vi "Tx to UDP.vi"(5 "Data Conversion":T1, 7 "Header Info":bool[](array[boolean]), 8 "error in (no error)":errorcluster, 9 "Byte Order":T4(ring), 10 "Tx Array":dbl[](array[numeric]), 11 "Packet ID":i32) -> (0 "error out":errorcluster, 2 "Tx String":string)   [LabVIEW 2016, in "UDP-Custom-Device Engine.lvlib"]
uses:
  UDP-Custom-Device Engine.lvlib
  Data Conversion Config.ctl
  <vilib>/NI Veristand/VeriStand Data/Library/Byte Buffer/Byte Buffer.lvclass
  <vilib>/NI Veristand/VeriStand Data/Library/Byte Buffer/Byte Buffer.Mapping.ctl
  <vilib>/NI Veristand/VeriStand Data/Library/Typedefs/Typedefs.Data Types.ctl
  <vilib>/NI Veristand/VeriStand Data/Library/Byte Buffer/Byte Buffer.lvclass/Byte Buffer.ctl
  <vilib>/NI Veristand/VeriStand Data/Library/Memory Management/Memory Management.MoveDblBlock.Write (Double).vi
  <vilib>/NI Veristand/VeriStand Data/Library/Byte Buffer/Byte Buffer.Write.Typed Array.vi
  <vilib>/NI Veristand/VeriStand Data/Library/Utilities/Utilities.Buffer.Double.vi
  <vilib>/NI Veristand/VeriStand Data/Library/Byte Buffer/Byte Buffer.Write.vi
  <vilib>/NI Veristand/VeriStand Data/Library/Byte Buffer/Byte Buffer.Write (1D Boolean).vi
  <vilib>/NI Veristand/VeriStand Data/Library/Type Conversion/Type Conversion.From Double.Subset.vi
  <vilib>/NI Veristand/VeriStand Data/Library/Type Conversion/Type Conversion.From Double.Subset (1D Boolean).vi
  <vilib>/NI Veristand/VeriStand Data/Library/Byte Buffer/Byte Buffer.Write (1D SGL).vi
  <vilib>/NI Veristand/VeriStand Data/Library/Type Conversion/Type Conversion.From Double.Subset (1D SGL).vi
  <vilib>/NI Veristand/VeriStand Data/Library/Byte Buffer/Byte Buffer.Write (1D DBL).vi
  <vilib>/NI Veristand/VeriStand Data/Library/Byte Buffer/Byte Buffer.Write (1D I8).vi
  <vilib>/NI Veristand/VeriStand Data/Library/Type Conversion/Type Conversion.From Double.Subset (1D I8).vi
  <vilib>/NI Veristand/VeriStand Data/Library/Byte Buffer/Byte Buffer.Write (1D I16).vi
  <vilib>/NI Veristand/VeriStand Data/Library/Type Conversion/Type Conversion.From Double.Subset (1D I16).vi
  <vilib>/NI Veristand/VeriStand Data/Library/Byte Buffer/Byte Buffer.Write (1D I32).vi
  <vilib>/NI Veristand/VeriStand Data/Library/Type Conversion/Type Conversion.From Double.Subset (1D I32).vi
  <vilib>/NI Veristand/VeriStand Data/Library/Byte Buffer/Byte Buffer.Write (1D I64).vi
  <vilib>/NI Veristand/VeriStand Data/Library/Type Conversion/Type Conversion.From Double.Subset (1D I64).vi
  <vilib>/NI Veristand/VeriStand Data/Library/Byte Buffer/Byte Buffer.Write (1D U8).vi
  <vilib>/NI Veristand/VeriStand Data/Library/Type Conversion/Type Conversion.From Double.Subset (1D U8).vi
  <vilib>/NI Veristand/VeriStand Data/Library/Byte Buffer/Byte Buffer.Write (1D U16).vi
  <vilib>/NI Veristand/VeriStand Data/Library/Type Conversion/Type Conversion.From Double.Subset (1D U16).vi
  <vilib>/NI Veristand/VeriStand Data/Library/Byte Buffer/Byte Buffer.Write (1D U32).vi
  <vilib>/NI Veristand/VeriStand Data/Library/Type Conversion/Type Conversion.From Double.Subset (1D U32).vi
  <vilib>/NI Veristand/VeriStand Data/Library/Byte Buffer/Byte Buffer.Write (1D U64).vi
  <vilib>/NI Veristand/VeriStand Data/Library/Type Conversion/Type Conversion.From Double.Subset (1D U64).vi
  <vilib>/NI Veristand/VeriStand Data/Library/Utilities/Utilities.Sizeof.Array.vi
  <vilib>/NI Veristand/VeriStand Data/Library/Type Conversion/Type Conversion.From Double.vi
  <vilib>/NI Veristand/VeriStand Data/Library/Type Conversion/Type Conversion.From Double (1D Boolean).vi
  <vilib>/NI Veristand/VeriStand Data/Library/Type Conversion/Type Conversion.From Double (1D SGL).vi
  <vilib>/NI Veristand/VeriStand Data/Library/Type Conversion/Type Conversion.From Double (1D I8).vi
  <vilib>/NI Veristand/VeriStand Data/Library/Type Conversion/Type Conversion.From Double (1D I16).vi
  <vilib>/NI Veristand/VeriStand Data/Library/Type Conversion/Type Conversion.From Double (1D I32).vi
  <vilib>/NI Veristand/VeriStand Data/Library/Type Conversion/Type Conversion.From Double (1D I64).vi
  <vilib>/NI Veristand/VeriStand Data/Library/Type Conversion/Type Conversion.From Double (1D U8).vi
  <vilib>/NI Veristand/VeriStand Data/Library/Type Conversion/Type Conversion.From Double (1D U16).vi
  <vilib>/NI Veristand/VeriStand Data/Library/Type Conversion/Type Conversion.From Double (1D U32).vi
  <vilib>/NI Veristand/VeriStand Data/Library/Type Conversion/Type Conversion.From Double (1D U64).vi
  <vilib>/NI Veristand/VeriStand Data/Library/Utilities/Utilities.Sizeof.Scalar.vi
  <vilib>/NI Veristand/VeriStand Data/Library/Memory Management/Memory Management.Handle Return.vi
  <vilib>/NI Veristand/VeriStand Data/Library/VeriStand Data.lvlib
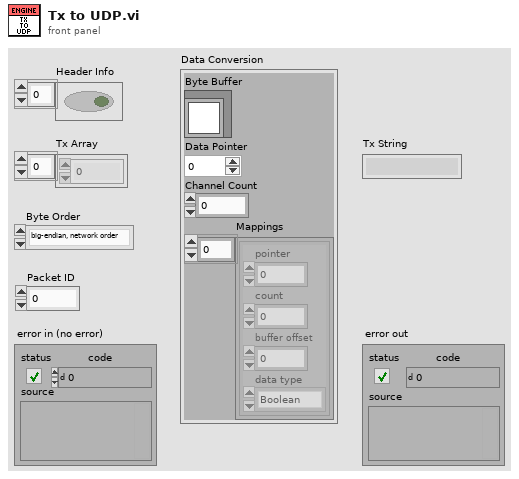
[diagram p1: front panel]
types:
  T1 = typedef "UDP-Custom-Device Engine.lvlib/Data Conversion Config.ctl" = cluster{"Byte Buffer":refnum<class "Byte Buffer.lvclass">, "Data Pointer":u64, "Channel Count":i32, "Mappings":T2[]}
  T2 = typedef "VeriStand Data.lvlib/Byte Buffer.lvclass/Byte Buffer.Mapping.ctl" = cluster{"pointer":u64, "count":i32, "buffer offset":i32, "data type":T3}
  T3 = typedef "VeriStand Data.lvlib/Typedefs.Data Types.ctl" = enum16{"Boolean", "Single", "Double", "I8", "I16", "I32", "I64", "U8", "U16", "U32", "U64"}
  T4 = enum16{"big-endian, network order", "native, host order", "little-endian"}
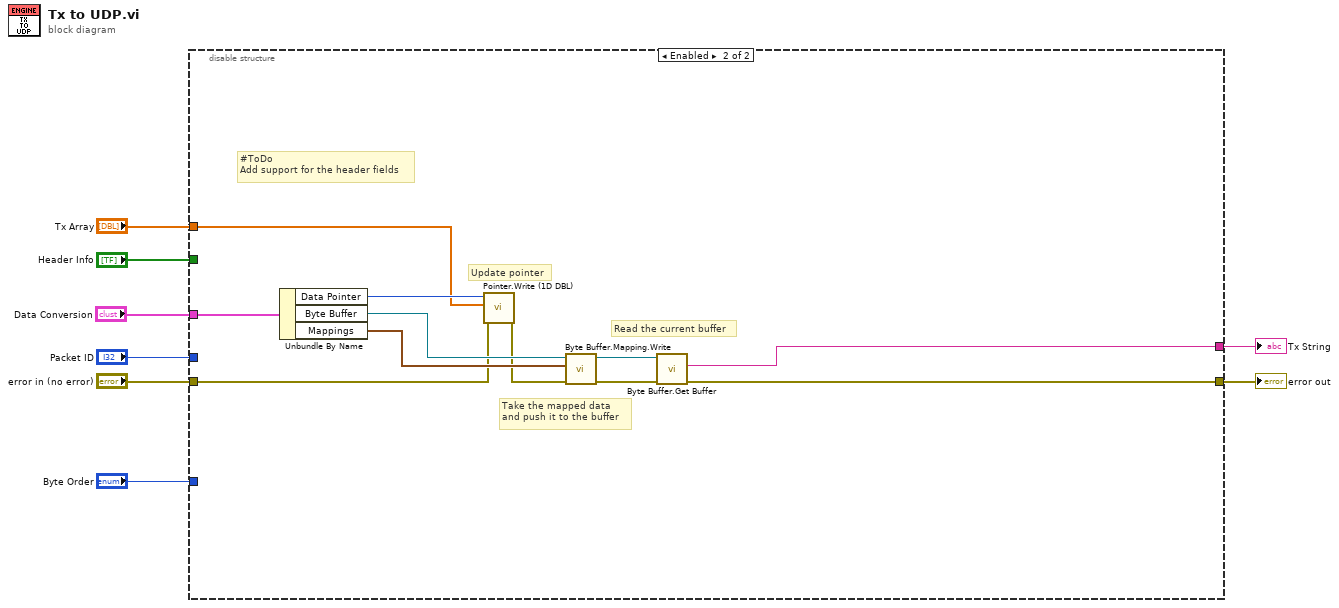
[diagram p0: block diagram]
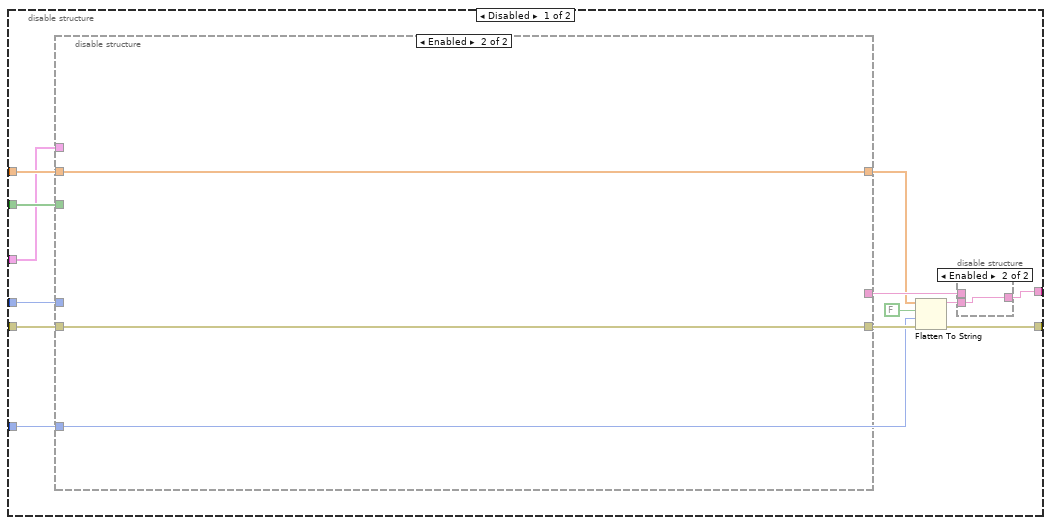
[diagram p2: hidden frame]
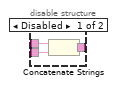
[diagram p3: hidden frame]
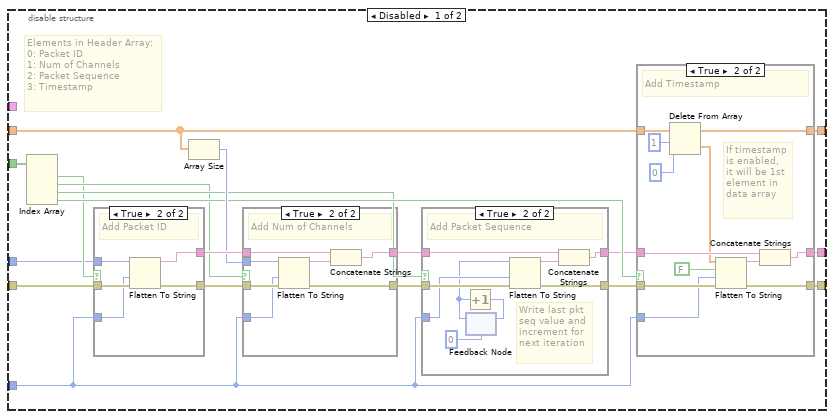
[diagram p4: hidden frame]
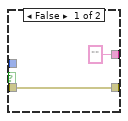
[diagram p8: hidden frame]
diagram:
  n1 = disable-structure shown="Enabled" {
    disable-tunnel: "error in (no error)" -> [w21 w94]
    disable-tunnel: [w20 w90] -> w7
    disable-tunnel: "Byte Order" -> [w16 _]
    disable-tunnel: "Header Info" -> [w15 _]
    disable-tunnel: "Tx Array" -> [w13 w97]
    disable-tunnel: "Packet ID" -> [w12 _]
    disable-tunnel: [w10 w89] -> w2
    disable-tunnel: "Data Conversion" -> [w9 w99]
    frame Disabled {
      n2 = disable-structure shown="Enabled" {
        disable-tunnel: w21 -> [w44 w87]
        disable-tunnel: [w40 w87] -> w17
        disable-tunnel: w16 -> [w38 _]
        disable-tunnel: w15 -> [w36 _]
        disable-tunnel: [w29 _] -> w14
        disable-tunnel: w13 -> [w28 w88]
        disable-tunnel: [w27 w88] -> w11
        disable-tunnel: w12 -> [w26 _]
        disable-tunnel: w9 -> [_ _]
        frame Disabled {
          # "Elements in Header Array:\n0: Packet ID\n1: Num of Channels\n2: Packet Sequence\n3: Timestamp"
          n3 = Index Array(array=w36) -> (element #1=w32:bool, element #2=w33:bool, element #3=w34:bool, element #4=w35:bool)  [unwired: 4 in]
          n4 = case shown="True" w32 {
            tunnel: w44 -> [w81 w86]
            tunnel: [w81 w85] -> w43
            tunnel: ["" ("data string") w84] -> w39
            tunnel: w38 -> [_ w83]
            tunnel: w26 -> [_ w82]
            frame False {
            }
            frame True {
              # "Add Packet ID"
              n5 = Flatten To String(anything=w82, byte order (0:big-endian, network order)=w83, error in (no error)=w86) -> (data string=w84:string, error out=w85:errorcluster)  [unwired: 1 in, 1 out]
            }
          }
          n6 = Array Size(array=w28) -> (size(s)=w37:i32)
          n7 = case shown="True" w33 {
            tunnel: w43 -> [w71 w79]
            tunnel: [w71 w78] -> w42
            tunnel: [w72 w75] -> w31
            tunnel: w38 -> [_ w76]
            tunnel: w39 -> [w72 w74]
            tunnel: w37 -> [_ w73]
            frame False {
            }
            frame True {
              # "Add Num of Channels"
              n8 = Flatten To String(anything=w73, byte order (0:big-endian, network order)=w76, error in (no error)=w79) -> (data string=w77:string, error out=w78:errorcluster)  [unwired: 1 in, 1 out]
              n9 = Concatenate Strings(w74, w77) -> (w75:string)
            }
          }
          n10 = case shown="True" w34 {
            tunnel: w42 -> [w60 w70]
            tunnel: [w60 w69] -> w41
            tunnel: [w61 w65] -> w30
            tunnel: w38 -> [_ w68]
            tunnel: w31 -> [w61 w67]
            frame False {
            }
            frame True {
              # "Write last pkt\nseq value and\nincrement for\nnext iteration"
              # "Add Packet Sequence"
              n11 = feedback #1(u64 0 ("Packet Sequence")) -> (w62:u64)
              n12 = Increment(x=w62) -> (x+1=w63:u64)
              n13 = feedback-in #1(w63) -> ()
              n14 = Flatten To String(anything=w62, byte order (0:big-endian, network order)=w68, error in (no error)=w70) -> (data string=w66:string, error out=w69:errorcluster)  [unwired: 1 in, 1 out]
              n15 = Concatenate Strings(w67, w66) -> (w65:string)
            }
          }
          n16 = case shown="True" w35 {
            tunnel: w41 -> [w46 w59]
            tunnel: [w46 w58] -> w40
            tunnel: [w47 w55] -> w29
            tunnel: w38 -> [_ w57]
            tunnel: w30 -> [w47 w54]
            tunnel: w28 -> [w45 w53]
            tunnel: [w45 w52] -> w27
            frame False {
            }
            frame True {
              # "If timestamp\nis enabled,\nit will be 1st\nelement in\ndata array"
              # "Add Timestamp"
              n17 = Delete From Array(array=w53, length=1, index=0) -> (deleted portion=w49:dbl[], array with subset deleted=w52:dbl[])
              n18 = Flatten To String(anything=w49, prepend array or string size? (T)=FALSE, byte order (0:big-endian, network order)=w57, error in (no error)=w59) -> (data string=w56:string, error out=w58:errorcluster)  [unwired: 1 out]
              n19 = Concatenate Strings(w54, w56) -> (w55:string)
            }
          }
        }
        frame Enabled {
        }
      }
      n20 = Flatten To String(anything=w11, prepend array or string size? (T)=FALSE, byte order (0:big-endian, network order)=w16, error in (no error)=w17) -> (data string=w19:string, error out=w20:errorcluster)  [unwired: 1 out]
      n21 = disable-structure shown="Enabled" {
        disable-tunnel: w19 -> [w24 w25]
        disable-tunnel: w14 -> [w23 _]
        disable-tunnel: [w22 w25] -> w10
        frame Disabled {
          n22 = Concatenate Strings(w23, w24) -> (w22:string)
        }
        frame Enabled {
        }
      }
    }
    frame Enabled {
      # "Read the current buffer"
      # "Take the mapped data\nand push it to the buffer"
      # "Update pointer"
      # "#ToDo\nAdd support for the header fields"
      n23 = Unbundle By Name(w99) -> ("Data Pointer"=w98:u64, "Byte Buffer"=w95:refnum<class "Byte Buffer.lvclass">, "Mappings"=w96:T2[])
      n24 = call <vilib>:"Pointer.Write (1D DBL).vi"("error in (no error)"=w94, "values"=w97, "pointer in"=w98) -> ("error out"=w93:errorcluster)  [unwired: 6 in, 2 out]
      n25 = call <vilib>:"Byte Buffer.Mapping.Write.vi"("error in (no error)"=w93, "mappings"=w96, "Byte Buffer in"=w95) -> ("error out"=w91:errorcluster, "Byte Buffer out"=w92:refnum<class "Byte Buffer.lvclass">)  [unwired: 6 in, 1 out]
      n26 = call <vilib>:"Byte Buffer.Get Buffer.vi"("error in (no error)"=w91, "Byte Buffer in"=w92) -> ("error out"=w90:errorcluster, "buffer"=w89:string)  [unwired: 7 in, 1 out]
    }
  }
  "error out" <- w7
  "Tx String" <- w2
